vi "Set Threshold Template.vi"(7 "Callback Option (off)":T1, 8 "error in (no error)":errorcluster, 9 "max":i16, 10 "min":i16, 11 "Template in":refnum<class "Template.lvclass">) -> (0 "error out":errorcluster, 3 "Template out":refnum<class "Template.lvclass">)   [LabVIEW 2011, in "Tinkerforge.lvlib" / "Template.lvclass"]
doc: "This VI sets the threshold configuration of the $FunctionName$."
uses:
  Template.lvclass
  Device/Type Definitions/Callback Option.ctl
  Device/Device.lvclass
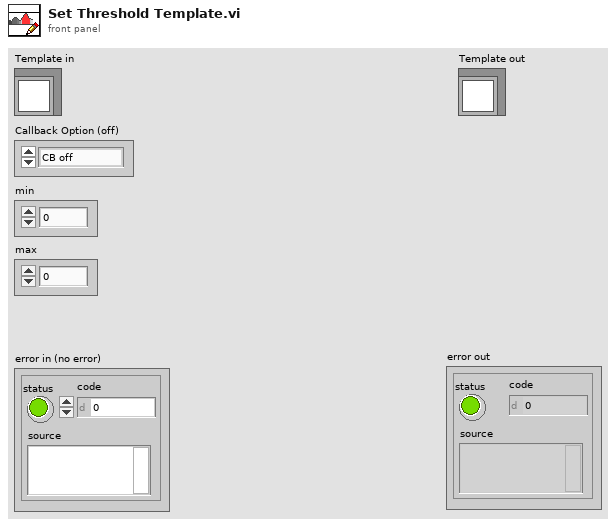
[diagram p1: front panel]
types:
  T1 = typedef "Tinkerforge.lvlib/Device.lvclass/Callback Option.ctl" = enum8{"CB off", "outside range", "inside range", "smaller", "greater"}
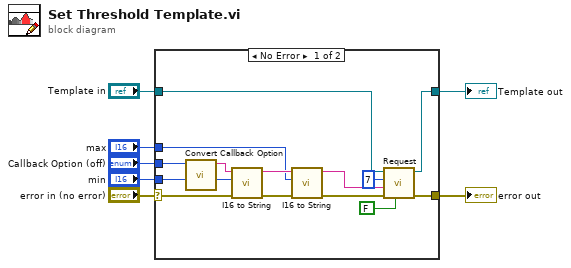
[diagram p0: block diagram]
diagram:
  n1 = case shown="No Error" "error in (no error)" {
    selector: "error in (no error)" -> [w15 w23]
    tunnel: [w17 w23] -> w6
    tunnel: [w20 w22] -> w4
    tunnel: "Template in" -> [w21 w22]
    tunnel: "min" -> [w14 _]
    tunnel: "max" -> [w10 _]
    tunnel: "Callback Option (off)" -> [w16 _]
    frame No Error {
      n2 = call "Convert Callback Option.vi"("Callback Option"=w16) -> ("Callback Option String"=w13:string)  [unwired: 10 in]
      n3 = call "I16 to String.vi"("Error In"=w15, "I16"=w14, "String in"=w13) -> ("Error Out"=w12:errorcluster, "String out"=w11:string)  [unwired: 7 in]
      n4 = call "I16 to String.vi"("Error In"=w12, "I16"=w10, "String in"=w11) -> ("Error Out"=w9:errorcluster, "String out"=w8:string)  [unwired: 7 in]
      n5 = call "Request.vi"("Response"=FALSE, "error in (no error)"=w9, "Data"=w8, "Function ID"=u8 7, "Device in"=w21) -> ("error out"=w17:errorcluster, "Device out"=w20:refnum<class "Template.lvclass">)  [unwired: 2 in, 3 out]
    }
    frame Error {
    }
  }
  "error out" <- w6
  "Template out" <- w4
